vi "Communication to Errors Handler.vi"(8 "error in":errorcluster) -> (0 "error out":errorcluster)   [LabVIEW 2020, in "ErrorHandler.lvlib"]
doc: "Uses the communication Manager FGV, to send a message to a module using one of its queue references"
uses:
  ErrorHandler.lvlib
  Controls/Error QMsg.ctl
  Support/Controls/Project Modules.ctl
  Support/Support.lvlib
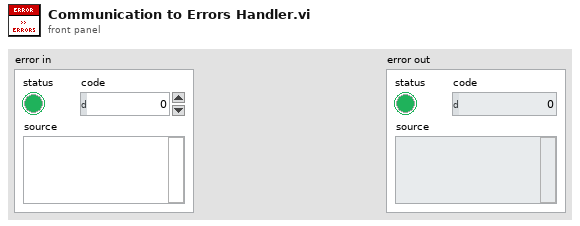
[diagram p1: front panel]
types:
  T1 = typedef "ErrorHandler.lvlib/Error QMsg.ctl" = cluster{"Command":string, "Data":errorcluster, "Source Module":T2}
  T2 = typedef "Support.lvlib/Project Modules.ctl" = enum16{"Controller", "Error", "Configuration Database", "Sensor Interface", "User Console", "Display Console"}
  T3 = typedef "ErrorHandler.lvlib/Module Messaging Structures.ctl" = cluster{">>EventHandlers":refnum<user-event>, ">>ErrorQ":refnum<queue>, ">>ControllerQ":refnum<queue>}
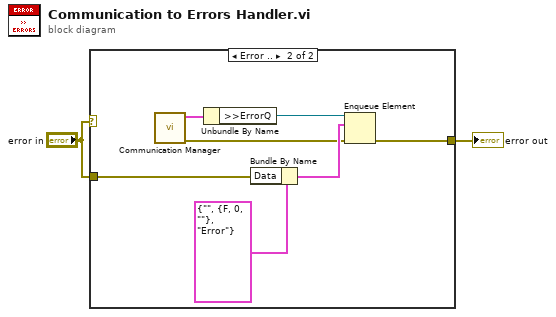
[diagram p0: block diagram]
diagram:
  n1 = case shown="Error .." "error in" {
    tunnel: "error in" -> [w3 w4]
    tunnel: [w3 w8] -> w1
    frame No Error {
    }
    frame Error {
      n2 = call "Communication Manager.vi"() -> ("error out"=w5:errorcluster, "Messaging Structures"=w10:T3)  [unwired: 10 in]
      n3 = Unbundle By Name(w10) -> (">>ErrorQ"=w9:refnum<queue>)
      n4 = Bundle By Name(cluster=T1 {"Command"="", "Data"={"status"=FALSE, "code"=0, "source"=""}, "Source Module"=enum."Error"} ("element"), "Data"=w4) -> (w6:T1)
      n5 = Enqueue Element(queue=w9, element=w6, error in (no error)=w5) -> (error out=w8:errorcluster)  [unwired: 1 in, 2 out]
    }
  }
  "error out" <- w1
